vi "GetPicture.vi"(8 "error in (no error)":errorcluster, 11 "DotNETCam in":refnum<class "DotNETCam.lvclass">) -> (0 "error out":errorcluster, 2 "2D Picture":picture, 3 "DotNETCam out":refnum<class "DotNETCam.lvclass">)   [LabVIEW 2021, in "DotNETCam.lvclass"]
uses:
  DotNETCam.lvclass
  C:/Localdata/Projects/TriekselSoft/TriekselsoftApplicationFramework/Source/.Externals/Library_YAF/YActor/YActor.lvclass
  .Externals/Library_YAF/YActor/YActor.lvclass/YActor.ctl
  .Externals/Library_YAF/YActor/ExeCmd_sync.vi
  788cf652-cfa8-44ab-bf5d-4ff5bf462e4f.vi
  .Externals/Library_YAF/YActor/private/SendCommand.vi
  .Externals/Library_YAF/YActor/private/WaitForReply.vi
  .Externals/Library_YAF/YActor/private/CreateLocalVI.vi
  .Externals/Library_YAF/YActor/private/ExeuteInlineVI.vi
  .Externals/Library_YAF/YActor/private/GetRemoteVIRef.vi
  .Externals/Library_YAF/YActor/private/GetNameOfVI.vi
  .Externals/Library_YAF/YActor/QuickCast.vi
  .Externals/Library_YAF/YActor/private/VINameProperty.vi
  .Externals/Library_YAF/YActor/private/MessageCounter.vi
  .Externals/Library_YAF/YActor/InlineReferencePool.vi
  .Externals/Library_YAF/YActor/private/ExecuteVI.vi
  .Externals/Library_YAF/YActor/YActor.lvclass
  C:/Localdata/Projects/TriekselSoft/TriekselsoftApplicationFramework/Source/.Externals/Library_YAF/YAFTAF/YAFTAF.lvclass
  C:/Localdata/Projects/TriekselSoft/TriekselsoftApplicationFramework/Source/.Externals/Interface_UserInterface_IFrontPanel/IFrontPanel/IFrontPanel.lvclass
  C:/Localdata/Projects/TriekselSoft/TriekselsoftApplicationFramework/Source/IInterface/IInterface.lvclass
  C:/Localdata/Projects/TriekselSoft/TriekselsoftApplicationFramework/Source/.Externals/Interface_Object_ICreateDestroy/ICreateDestroy/ICreateDestroy.lvclass
  C:/Localdata/Projects/TriekselSoft/TriekselsoftApplicationFramework/Source/.Externals/Interface_Object_IPersistentData/IPersistentData/IPersistentData.lvclass
  C:/Localdata/Projects/TriekselSoft/TriekselsoftApplicationFramework/Source/.Externals/Interface_TAF_ITAFObject/ITAFObject/ITAFObject.lvclass
  C:/Localdata/Projects/TriekselSoft/TriekselsoftApplicationFramework/Source/YAFTAFObjects/DotNETCam/DotNETCam.lvclass
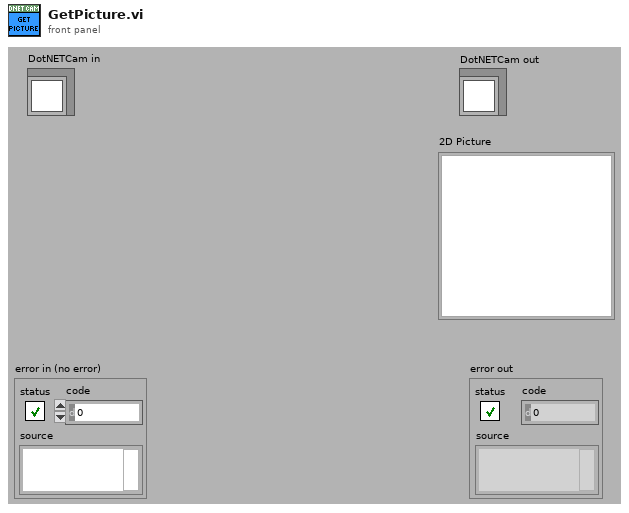
[diagram p1: front panel]
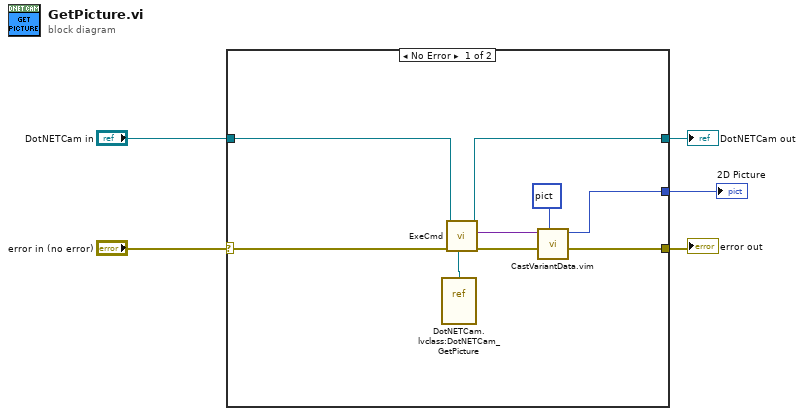
[diagram p0: block diagram]
diagram:
  n1 = case shown="No Error" "error in (no error)" {
    selector: "error in (no error)" -> [w13 w16]
    tunnel: [w9 w16] -> w4
    tunnel: [w11 w15] -> w2
    tunnel: "DotNETCam in" -> [w12 w15]
    tunnel: [w6 _] -> w1
    frame No Error {
      n2 = vi-ref "DotNETCam.lvclass:DotNETCam_GetPicture.vi"() -> (w14:refnum<vi>)
      n3 = call-poly "ExeCmd.vi"("CmdVIRef"=w14, "ErrorIn"=w13, "YActor in"=w12) -> ("ErrorOut"=w10:errorcluster, "ReplyData"=w8:variant, "YActor out"=w11:refnum<class "DotNETCam.lvclass">)  [unwired: 6 in]
      n4 = call "CastVariantData.vim"("Type"=picture data[5B] ("2D Picture"), "error in"=w10, "DataIn"=w8) -> ("error out"=w9:errorcluster, "DataOut"=w6:picture)  [unwired: 7 in]
    }
    frame Error {
    }
  }
  "error out" <- w4
  "DotNETCam out" <- w2
  "2D Picture" <- w1
